vi "Self Configure.vi"(8 "error in":errorcluster, 11 "Report in":refnum<class "Report.lvclass">) -> (0 "error out":errorcluster, 3 "Report out":refnum<class "Report.lvclass">)   [LabVIEW 2023, in "Report.lvlib" / "Report.lvclass"]
uses:
  Report.lvclass
  Report.lvclass/Report.ctl
  Accessors/Write Root Path.vi
  Accessors/Read Open.vi
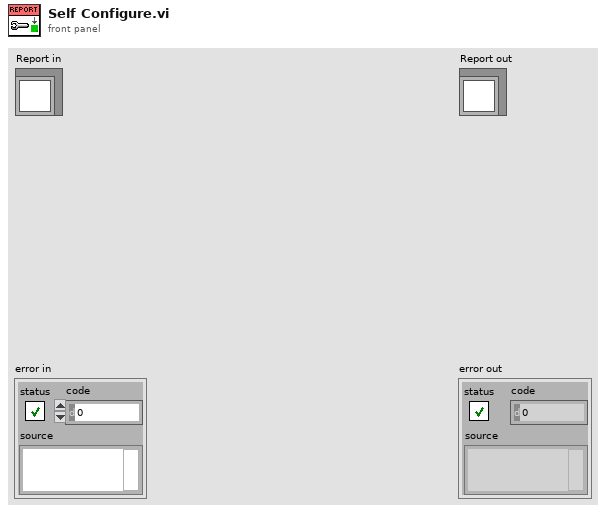
[diagram p1: front panel]
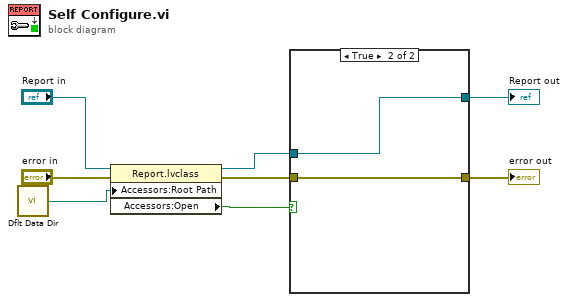
[diagram p0: block diagram]
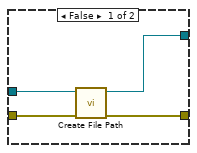
[diagram p2: hidden frame]
diagram:
  n1 = call <vilib>:"Dflt Data Dir.vi"() -> ("App:Default Data Directory"=w4:path)
  n2 = property class="Report.lvclass"(reference="Report in", error in="error in", "Accessors:Root Path"=w4) -> (reference out=w5:refnum<class "Report.lvclass">, error out=w1:errorcluster, "Accessors:Open"=w3:bool)
  n3 = case shown="True" w3 {
    tunnel: w5 -> [w12 w14]
    tunnel: [w11 w14] -> w8
    tunnel: [w10 w13] -> w7
    tunnel: w1 -> [w9 w13]
    frame False {
      n4 = call "Create File Path.vi"("error in"=w9, "Report in"=w12) -> ("error out"=w10:errorcluster, "Report out"=w11:refnum<class "Report.lvclass">)  [unwired: 8 in]
    }
    frame True {
    }
  }
  "error out" <- w7
  "Report out" <- w8
